vi "Fetch Multi Eval Meas List Segment ES Flatness Subcarrier Index Results.vi"(7 "Segment (1)":T3=1, 8 "error in (no error)":errorcluster, 10 "Instance (1)":T4=1, 11 "VISA resource name":refnum<visa-resource-name>) -> (0 "error out":errorcluster, 1 "Subcarrier Index Results":T2, 2 "Reliability Results":T1, 3 "VISA resource name out":refnum<visa-resource-name>, 4 "Statistic Expired":i32, 5 "Out Of Tolerance":dbl format="%^.3e")   [LabVIEW 2015, in "Rohde&Schwarz CMXP NR FR2 Measurement.lvlib"]
doc: "Returns subcarrier indices of the equalizer spectrum flatness measurement for segment <no> in list mode. At these SC indices, the current minimum and maximum power of the equalizer coefficients have been detected within range 1 and range 2.\n\nAttribute:\nRSCMXPNRFR2M_ATTR_FETCH_MULTI_EVAL_MEASUREMENT_LIST_SEGMENT_ESF_SUBCARRIER_INDEX_RESULTS\n\nRemote-control command:\nFETCh:NRMMw:MEAS<i>:MEValuation:LIST:SEGMent<no>:ESFLatness:CURRent:SCINdex?"
uses:
  <instrlib>/Rohde&Schwarz CMXP NR FR2 Measurement/Rohde&Schwarz CMXP NR FR2 Measurement.lvlib
  <instrlib>/Rohde&Schwarz CMXP NR FR2 Measurement/Private/_Instance.ctl
  <instrlib>/Rohde&Schwarz CMXP NR FR2 Measurement/Private/_Segment.ctl
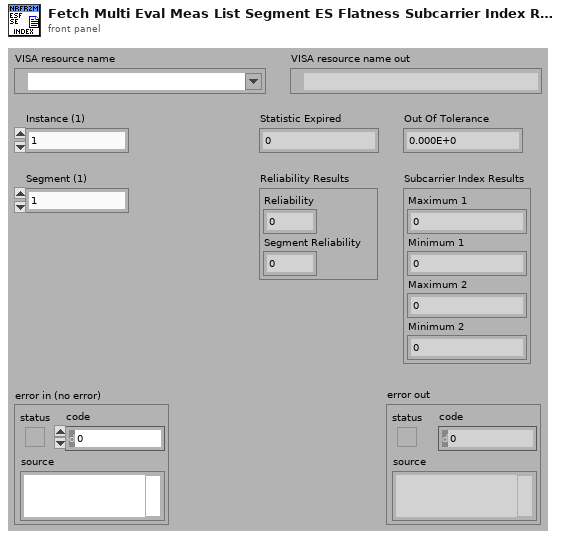
[diagram p1: front panel]
types:
  T1 = cluster{"Reliability":i32, "Segment Reliability":i32}
  T2 = cluster{"Maximum 1":i32, "Minimum 1":i32, "Maximum 2":i32, "Minimum 2":i32}
  T3 = typedef "Rohde&Schwarz CMXP NR FR2 Measurement.lvlib/_Segment.ctl" = i32
  T4 = typedef "Rohde&Schwarz CMXP NR FR2 Measurement.lvlib/_Instance.ctl" = i32
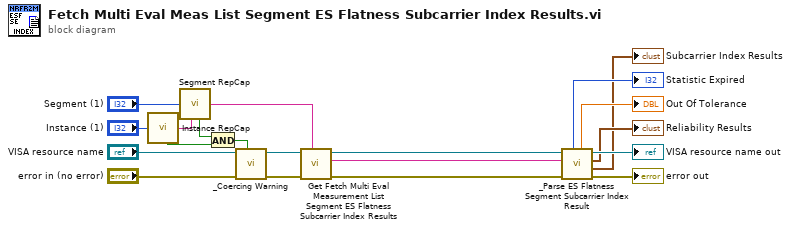
[diagram p0: block diagram]
diagram:
  n1 = call <instrlib>:"Instance RepCap.vi"("Instance In"="Instance (1)") -> ("In Range?"=w18:bool, "RepCap Identifier Out"=w1:string)  [unwired: 1 in]
  n2 = call <instrlib>:"Segment RepCap.vi"("Segment In"="Segment (1)", "RepCap String In (\"\")"=w1) -> ("In Range?"=w19:bool, "RepCap Identifier Out"=w3:string)
  n3 = And(x=w19, y=w18) -> (x .and. y?=w20:bool)
  n4 = call <instrlib>:"_Coercing Warning.vi"("In Range?"=w20, "error in (no error)"="error in (no error)", "VISA resource name"="VISA resource name") -> ("error out"=w13:errorcluster, "VISA resource name out"=w12:refnum<visa-resource-name>)  [unwired: 7 in]
  n5 = call "Get Fetch Multi Eval Measurement List Segment ES Flatness Subcarrier Index Results"("Repeated Capabilities"=w3, "error in (no error)"=w13, "instrument handle"=w12) -> ("error out"=w11:errorcluster, "Fetch Multi Eval Measurement List Segment ES Flatness Subcarrier Index Results"=w10:string, "instrument handle out"=w9:refnum<visa-resource-name>)  [unwired: 6 in]
  n6 = call <instrlib>:"_Parse ES Flatness Segment Subcarrier Index Result.vi"("error in (no error)"=w11, "Input String"=w10, "VISA resource name"=w9) -> ("error out"=→"error out":errorcluster, "Subcarrier Index Results"=→"Subcarrier Index Results":T2, "Reliability Results"=→"Reliability Results":T1, "VISA resource name out"=→"VISA resource name out":refnum<visa-resource-name>, "Out Of Tolerance"=→"Out Of Tolerance":dbl, "Statistic Expired"=→"Statistic Expired":i32)  [unwired: 3 in]
